vi "Robotic_Arm_Simulation.vi"() -> ()   [LabVIEW 2014]
uses:
  <vilib>/Simulation/Scripting/Companion Diagram/SimConfigNode/SimParams.ctl
  <vilib>/Simulation/Scripting/Companion Diagram/SimConfigNode/_simSolvers.ctl
  <vilib>/Simulation/Implementation/Shared/SIMSCR Execution Mode.ctl
  <vilib>/Simulation/Param Hierarchy/Typedefs/SIMPH Param Control Actions.ctl
  <vilib>/Simulation/Implementation/Shared/NILVSim_ParamChanged.vi
  <vilib>/Simulation/Implementation/Shared/NILVSIM_BeginStep.vi
  <vilib>/Simulation/DataSources/Implementation/NILVSim Step.llb/SIM Step (scalar).vi
  <vilib>/Simulation/Utility/Implementation/NILVSim Collector.llb/SIM Collector (scalar).vi
  <vilib>/Simulation/SignalDisplay/Implementation/NILVSim Time Waveform.llb/SIM Time Waveform (scalar).vi
  <vilib>/Simulation/DiscreteLinear/Implementation/NILVSim Discrete Integrator Forward.llb/SIM Discrete Integrator Forward Distributor (scalar).vi
  <vilib>/Simulation/DiscreteLinear/Implementation/NILVSim Discrete Integrator Forward.llb/SIM Discrete Integrator Forward Collector (scalar).vi
  <vilib>/Simulation/Implementation/Shared/SIM Is Init or Final Stage.vi
  <vilib>/Simulation/SignalArithmetic/Implementation/NILVSim Gain.llb/SIM Gain (scalar).vi
  <vilib>/Simulation/Implementation/Shared/NILVSim_Manager.vi
  <vilib>/Utility/error.llb/Clear Errors.vi
  <vilib>/Simulation/Implementation/Shared/NILVSim_FinalizeModel.vi
  <vilib>/Simulation/Utility/Implementation/NILVSim Collector.llb/NILVSim Collector core (scalar).vi
  <vilib>/Simulation/Implementation/Shared/SIM Unbundle Sim Info.vi
  <vilib>/Simulation/Implementation/Shared/NILVSim_Initialize.vi
  <vilib>/Simulation/Utility/Implementation/NILVSim Get Time and IsAcceptedStep.vi
  <vilib>/addons/control/pid/pid.llb/PID.vi
  <vilib>/addons/control/pid/pid.llb/PID (DBL).vi
  <vilib>/Simulation/Implementation/Shared/SIMSH Read Queue.vi
  <vilib>/Simulation/Implementation/Shared/NILVSim_GetModelError.vi
  <vilib>/Simulation/Implementation/Shared/SIM Bundle Sim Info.vi
  <vilib>/Simulation/Scripting/Companion Diagram/SimConfigNode/SimDog.xnode
  <vilib>/Simulation/Implementation/XNodeFramework/SimXNode/SimX.xnode
  <vilib>/Simulation/EMI/Plugins/FMI for Model Exchange/EMI_FMIL.dll
  <vilib>/addons/control/pid/NI_PID_pid.lvlib
  <vilib>/Simulation/DiscreteLinear/Implementation/NILVSim Discrete Integrator Forward.llb/SIM Discrete Integrator Forward (scalar).vi
  <vilib>/Simulation/Implementation/Shared/NI_SIM_Implementation.lvlib
panel:
  out "Angular Velocity 3":cluster{"Time":dbl[], "Signal":dbl[]}(graph)
  out "Angle 3":cluster{"Time":dbl[], "Signal":dbl[]}(graph)
  out "Angular Velocity 2":cluster{"Time":dbl[], "Signal":dbl[]}(graph)
  out "Angle 2":cluster{"Time":dbl[], "Signal":dbl[]}(graph)
  out "Angular Velocity":cluster{"Time":dbl[], "Signal":dbl[]}(graph)
  out "Angle":cluster{"Time":dbl[], "Signal":dbl[]}(graph)
  out "Axis 3 Velocity":waveform(dbl)(graph)
  out "Axis 3 Position":waveform(dbl)(graph)
  out "Axis 2 Velocity":waveform(dbl)(graph)
  out "Axis 2 Position":waveform(dbl)(graph)
  out "Axis 1 Velocity":waveform(dbl)(graph)
  out "Axis 1 Position":waveform(dbl)(graph)
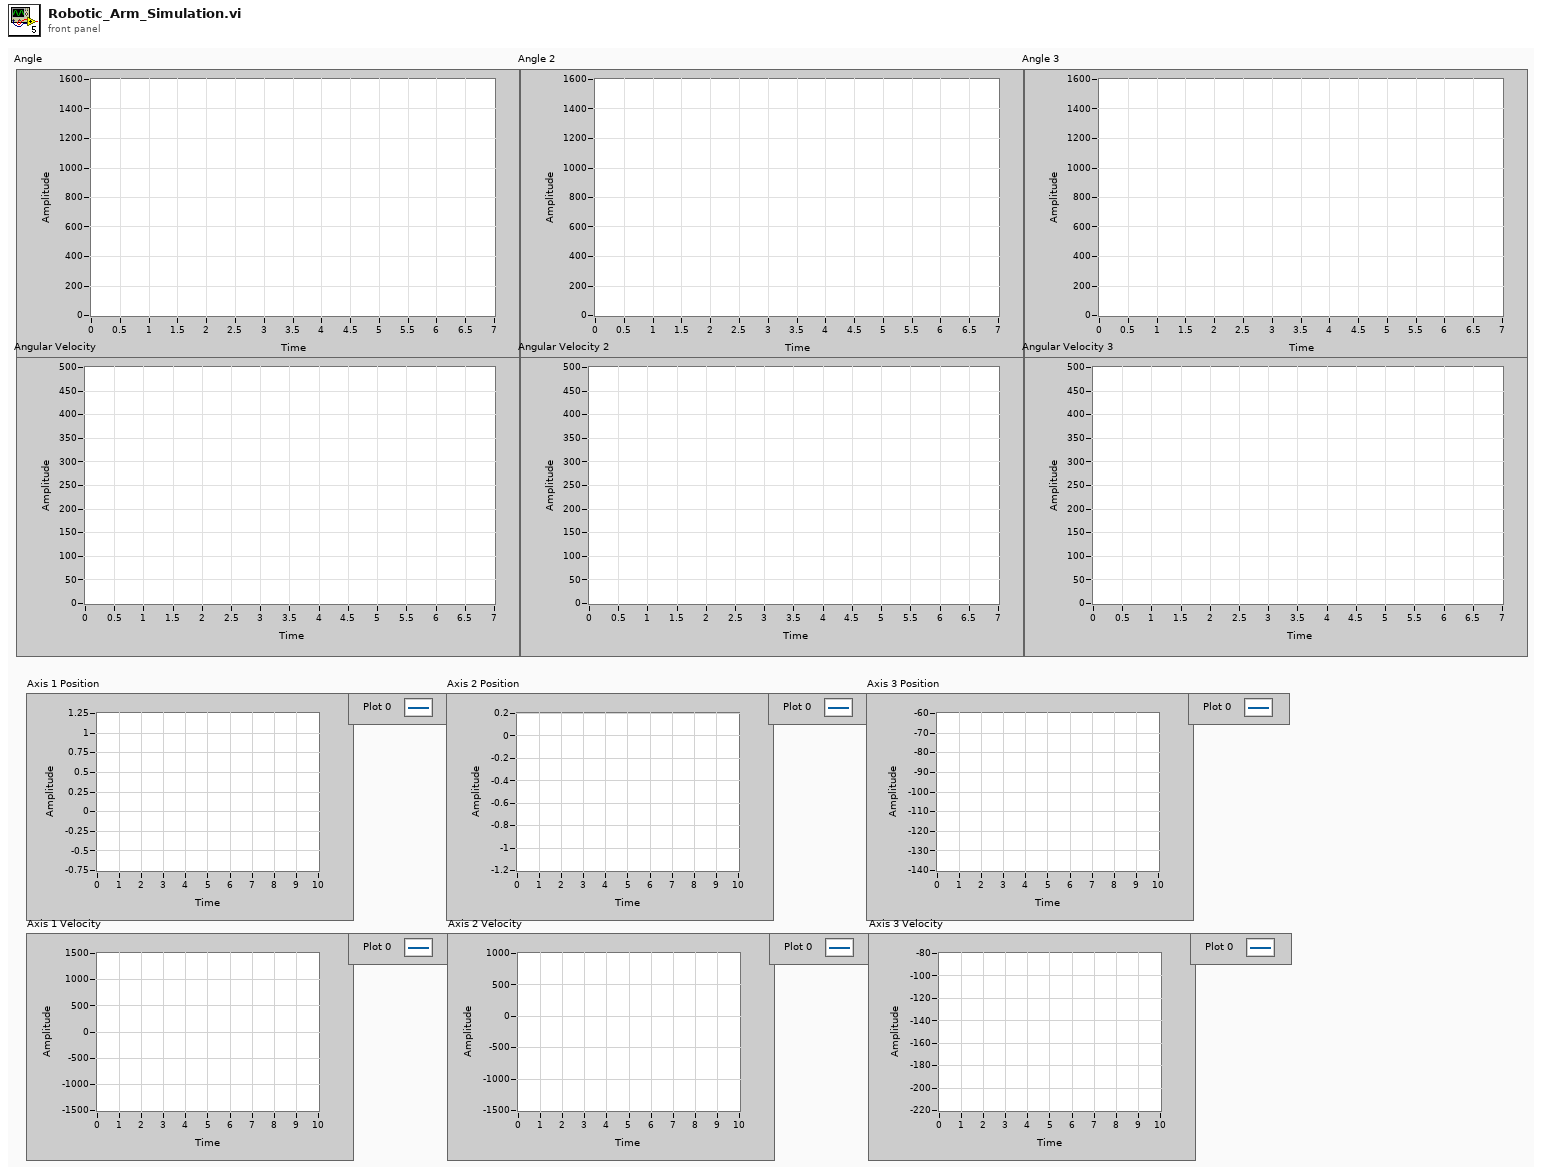
[diagram p1: front panel]
types:
  T1 = enum16{"Runge-Kutta 1 (Euler)", "Runge-Kutta 2", "Runge-Kutta 3", "Runge-Kutta 4", "Runge-Kutta 23 (variable)", "Runge-Kutta 45 (variable)", "BDF (variable)", "Adams-Moulton (variable)", "Rosenbrock (variable)", "Discrete States Only", "SDIRK 4 (variable)", "Radau 5 (variable)", "Radau 9 (variable)", "Radau 13 (variable)", "Radau [Variable Order] (variable)", "Gear's Method (variable)"}
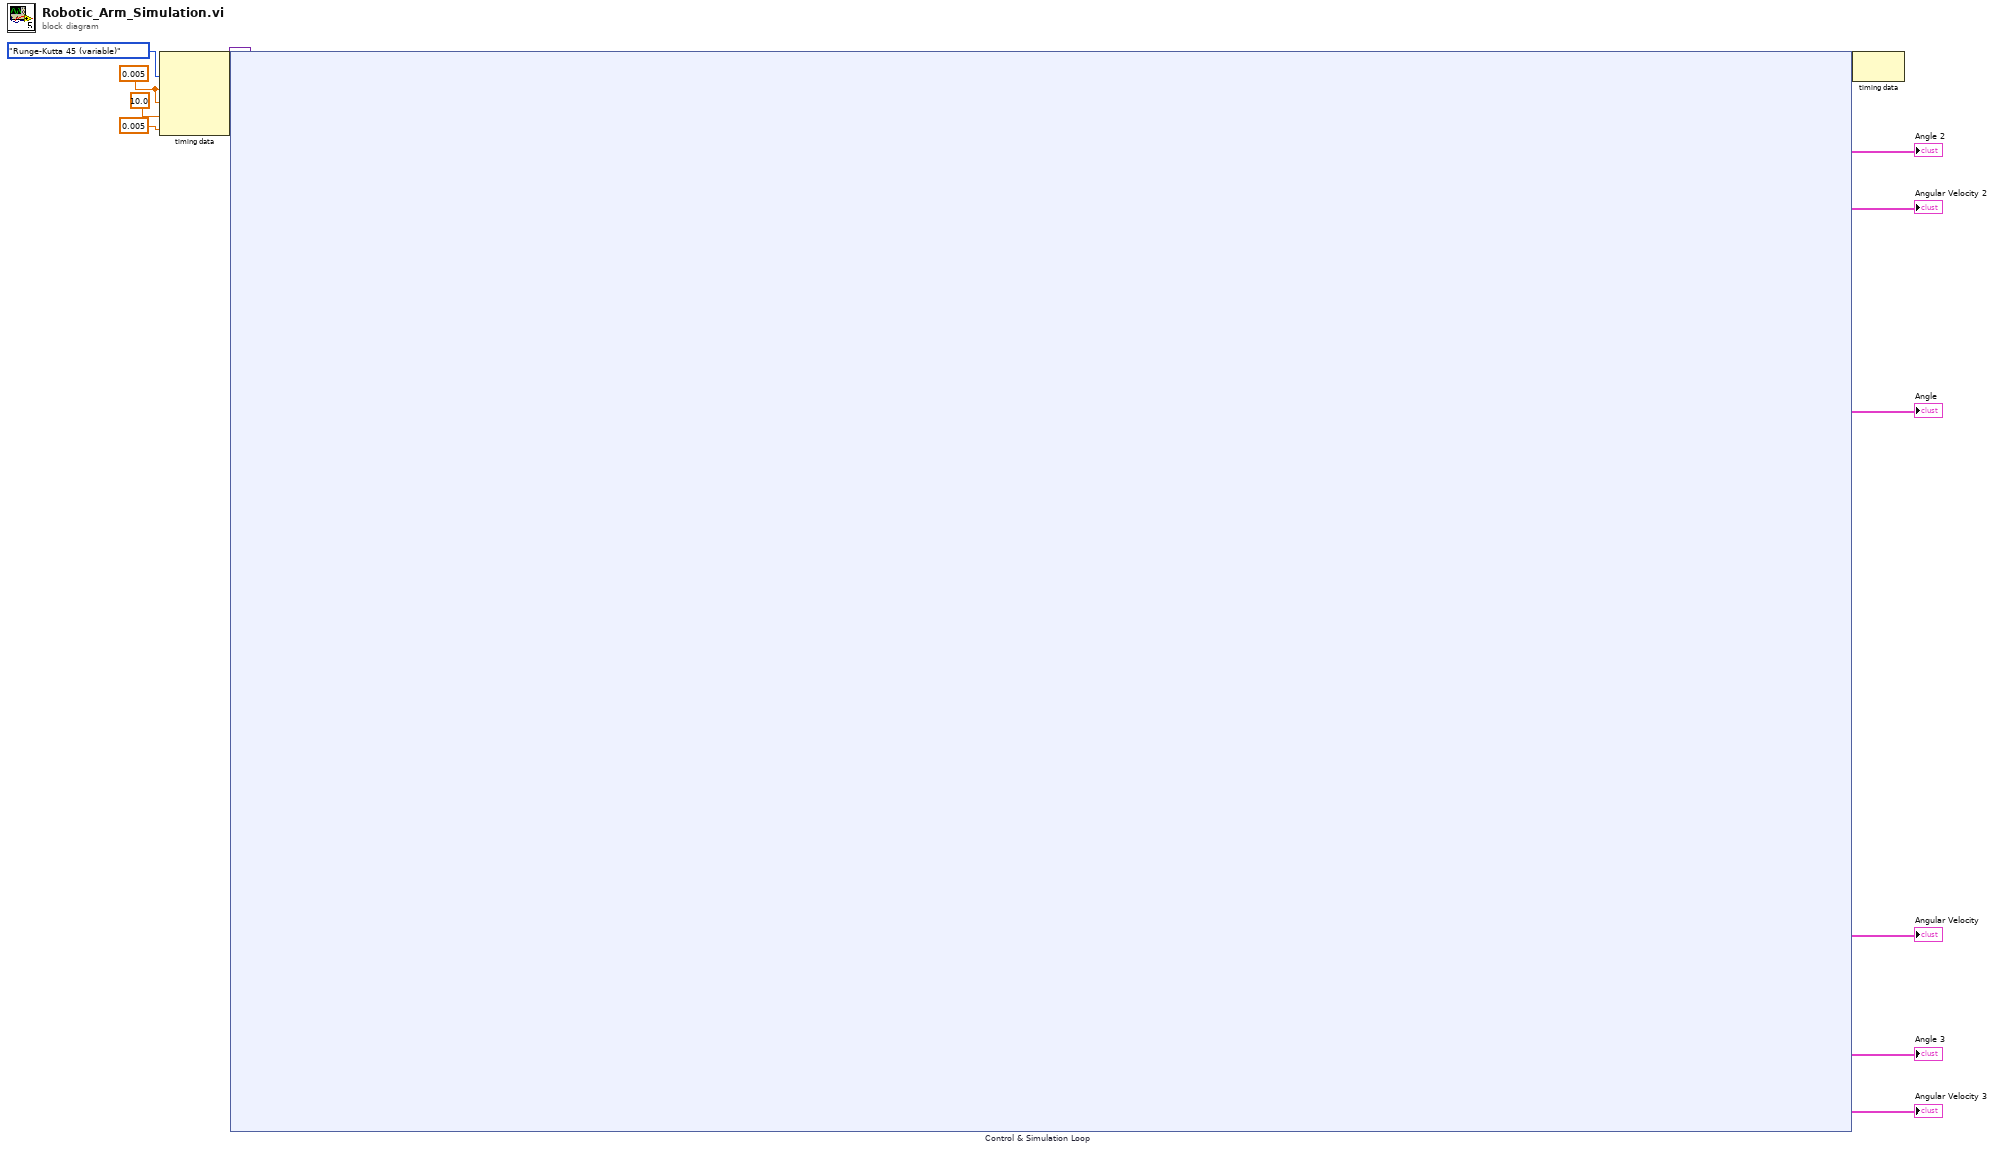
[diagram p0: block diagram]
diagram:
  w8 = 0.005 ("Maximum Step Size (s)")
  n1 = node-c288(T1."Runge-Kutta 45 (variable)" ("ODE Solver"), w8, w8, 10.0 ("Final Time (s)"), 0.005 ("Discrete Step Size (s)")) -> (w12:variant)
  n2 = node-c254 "Control & Simulation Loop"(w12) -> (w11:variant, →"Angle":cluster{"Time":dbl[], "Signal":dbl[]}, →"Angular Velocity":cluster{"Time":dbl[], "Signal":dbl[]}, →"Angle 2":cluster{"Time":dbl[], "Signal":dbl[]}, →"Angular Velocity 2":cluster{"Time":dbl[], "Signal":dbl[]}, →"Angle 3":cluster{"Time":dbl[], "Signal":dbl[]}, →"Angular Velocity 3":cluster{"Time":dbl[], "Signal":dbl[]})
  n3 = node-c288(w11) -> ()  [unwired: 1 out]
